vi "Read Controller queues.vi"(11 "Communication in":refnum<class "Communication.lvclass">) -> (2 "State command queues":refnum<queue>[](array[refnum]))   [LabVIEW 2024, in "Communication.lvclass"]
doc: "MIT Licence\nCopyright (c) 2024 David Grollier"
uses:
  Communication.lvclass
  Game Componants/Game Board/State Command.ctl
  Communication.lvclass/Communication.ctl
  Game Componants/Game Board/Game Board.lvclass
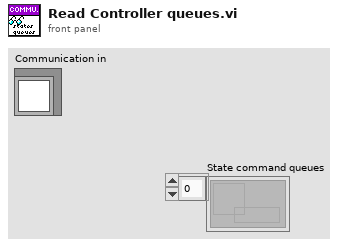
[diagram p1: front panel]
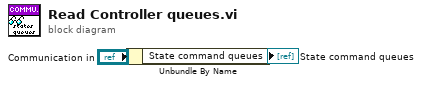
[diagram p0: block diagram]
diagram:
  n1 = Unbundle By Name("Communication in") -> ("State command queues"=→"State command queues":refnum<queue>[])
